vi "Initiate Trigger.vi"(8 "error in (no error)":errorcluster, 9 "Enable Continuous Transient Trigger (T: Enable)":bool=TRUE, 10 "Initiate System (0: Acquisition)":u16(ring) items=["Acquisition", "External Logging", "Transient"], 11 "VISA resource name":refnum<visa-resource-name>) -> (0 "error out":errorcluster, 3 "VISA resource name out":refnum<visa-resource-name>)   [LabVIEW 2021, in "Agilent N6900 N7900 Series.lvlib"]
doc: "Initiates the trigger system that is specified.\n\nNote:\nUse this VI only with other low-level VIs. The high-level VIs automatically incorporate this functionality. This VI does not check the instrument status."
uses:
  <instrlib>/Agilent N6900 N7900 Series/Agilent N6900 N7900 Series.lvlib
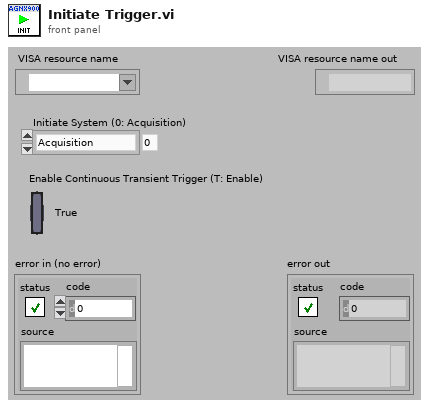
[diagram p1: front panel]
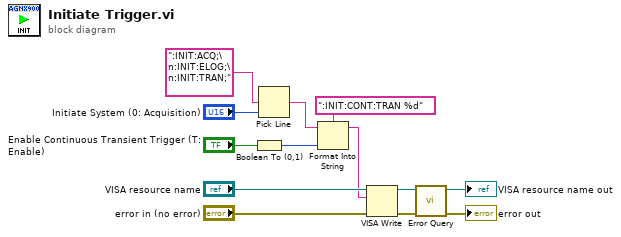
[diagram p0: block diagram]
diagram:
  n1 = Boolean To (0,1)(Boolean="Enable Continuous Transient Trigger (T: Enable)") -> (0, 1=w6:i16)
  n2 = Pick Line(multi-line string=":INIT:ACQ;\n:INIT:ELOG;\n:INIT:TRAN;" ("format string"), line index="Initiate System (0: Acquisition)") -> (output string=w4:string)  [unwired: 1 in]
  n3 = Format Into String(format string=":INIT:CONT:TRAN %d", initial string=w4, w6) -> (resulting string=w7:string)  [unwired: 1 in, 1 out]
  n4 = VISA Write(VISA resource name="VISA resource name", write buffer=w7, error in (no error)="error in (no error)") -> (VISA resource name out=w10:refnum<visa-resource-name>, error out=w11:errorcluster)  [unwired: 1 out]
  n5 = call <instrlib>:"Error Query.vi"("error in (no error)"=w11, "VISA resource name"=w10) -> ("error out"=→"error out":errorcluster, "VISA resource name out"=→"VISA resource name out":refnum<visa-resource-name>)  [unwired: 6 in, 2 out]
